vi "A3_ArquitectuaProductorConsumidor.vi"() -> ()   [LabVIEW 2025]
panel:
  in  "milliseconds to wait 2":u32
  in  "milliseconds to wait":u32
  in  "stop":bool
  out "Waveform Chart":dbl(graph)
  out "# elements in queue":i32
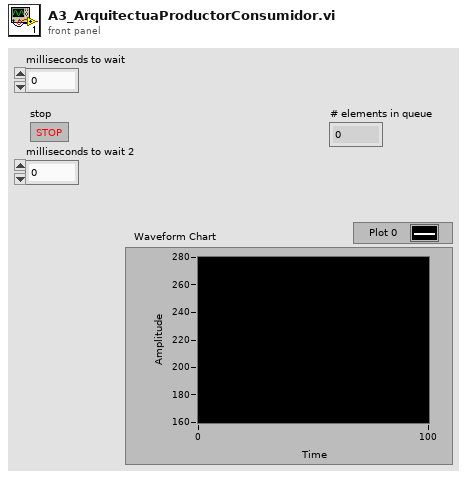
[diagram p1: front panel]
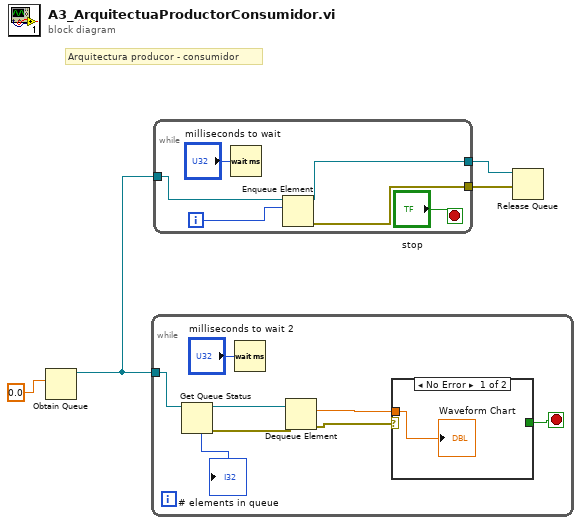
[diagram p0: block diagram]
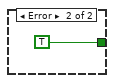
[diagram p2: hidden frame]
diagram:
  # "Arquitectura producor - consumidor"
  n1 = Obtain Queue(element data type=0.0) -> (queue out=w2:refnum<queue>)  [unwired: 4 in, 2 out]
  n2 = while {
    tunnel: w2 -> [w12]
    stop <- w6 stop-if-true
    n3 = Get Queue Status(queue=w12) -> (queue out=w11:refnum<queue>, error out=w10:errorcluster, # elements in queue=→"# elements in queue":i32)  [unwired: 2 in, 5 out]
    n4 = Wait (ms)(milliseconds to wait="milliseconds to wait 2") -> ()  [unwired: 1 out]
    n5 = Dequeue Element(queue=w11, error in (no error)=w10) -> (element=w7:dbl, error out=w8:errorcluster)  [unwired: 1 in, 2 out]
    n6 = case shown="No Error" w8 {
      tunnel: w7 -> [w13 _]
      tunnel: [_ TRUE] -> w6
      frame No Error {
        "Waveform Chart" <- w13
      }
      frame Error {
      }
    }
  }
  n7 = while {
    tunnel: [w19] -> w4
    tunnel: [w18] -> w3
    tunnel: w2 -> [w17]
    i -> [w20]
    stop <- "stop" stop-if-true
    n8 = Wait (ms)(milliseconds to wait="milliseconds to wait") -> ()  [unwired: 1 out]
    n9 = Enqueue Element(queue=w17, element=w20) -> (queue out=w18:refnum<queue>, error out=w19:errorcluster)  [unwired: 2 in, 1 out]
  }
  n10 = Release Queue(queue=w3, error in (no error)=w4) -> ()  [unwired: 1 in, 3 out]
